vi "Teleop.vi"(10 "Match Info":T2={"Autonomous Elapsed Seconds"=0.0, "TeleOp Elapsed Seconds"=0.0, "Disabled Elapsed Seconds"=0.0, "Visited Autonomous"=FALSE, "Visited TeleOp"=FALSE, "Visited Disabled"=FALSE, "Autonomous Settings"={"Autonomous Style"=enum."Independent", "VI Refnum"=refnum}}, 11 "Call Context":T3) -> ()   [LabVIEW 2023]
doc: "This VI is called for each TeleOp packet received from the DS where the robot is not disabled. It is often used to read from the joysticks and update I/O or to update setpoints for timed control loops. It should complete and return within 20 milliseconds or it may miss DS packets."
uses:
  <vilib>/Rock Robotics/WPI/DriverStation/WPI_DriverStationDerivedRobotMode.ctl
  <vilib>/Rock Robotics/WPI/DriverStation/WPI_DriverStationMatch Info.ctl
  Shared Code/TypeDefs/ENUM_CMD_Mode Select.ctl
  Teleop Support/ENUM_Axes Select.ctl
  Systems/SwerveDrive/Cluster_CMD_ACT_Data.ctl
  Shared Code/TypeDefs/Cluster_CMD_Direction Data.ctl
  Shared Code/TypeDefs/Cluster_Module Velocity-Direction-Rotations.ctl
  Shared Code/TypeDefs/Level_Velocity plus-minus 1.ctl
  Shared Code/TypeDefs/Dial_Compase heading unit circle CCW positive.ctl
  Shared Code/TypeDefs/Cluster_X-Y.ctl
  8b3177bb-dc82-4863-aed5-aa104a122ccc.vi
  83fdd1ca-84e3-4cf5-86f5-8b3c56b849f5.vi
  <vilib>/Rock Robotics/Network Tables/NT Write Boolean.vi
  Systems/Game Controller/Global_SEN_Data Out.vi
  Systems/SwerveDrive/Global_CMD_ACT_Data In.vi
  Systems/Game Controller/GameController_SEN.lvlib
  Systems/SwerveDrive/SwerveDrive_ACT_ts.lvlib
panel:
  in  "MAx Traverse Speed FPS Out":dbl=5.0
  out "Drive Mode":T1
  out "POV":i16
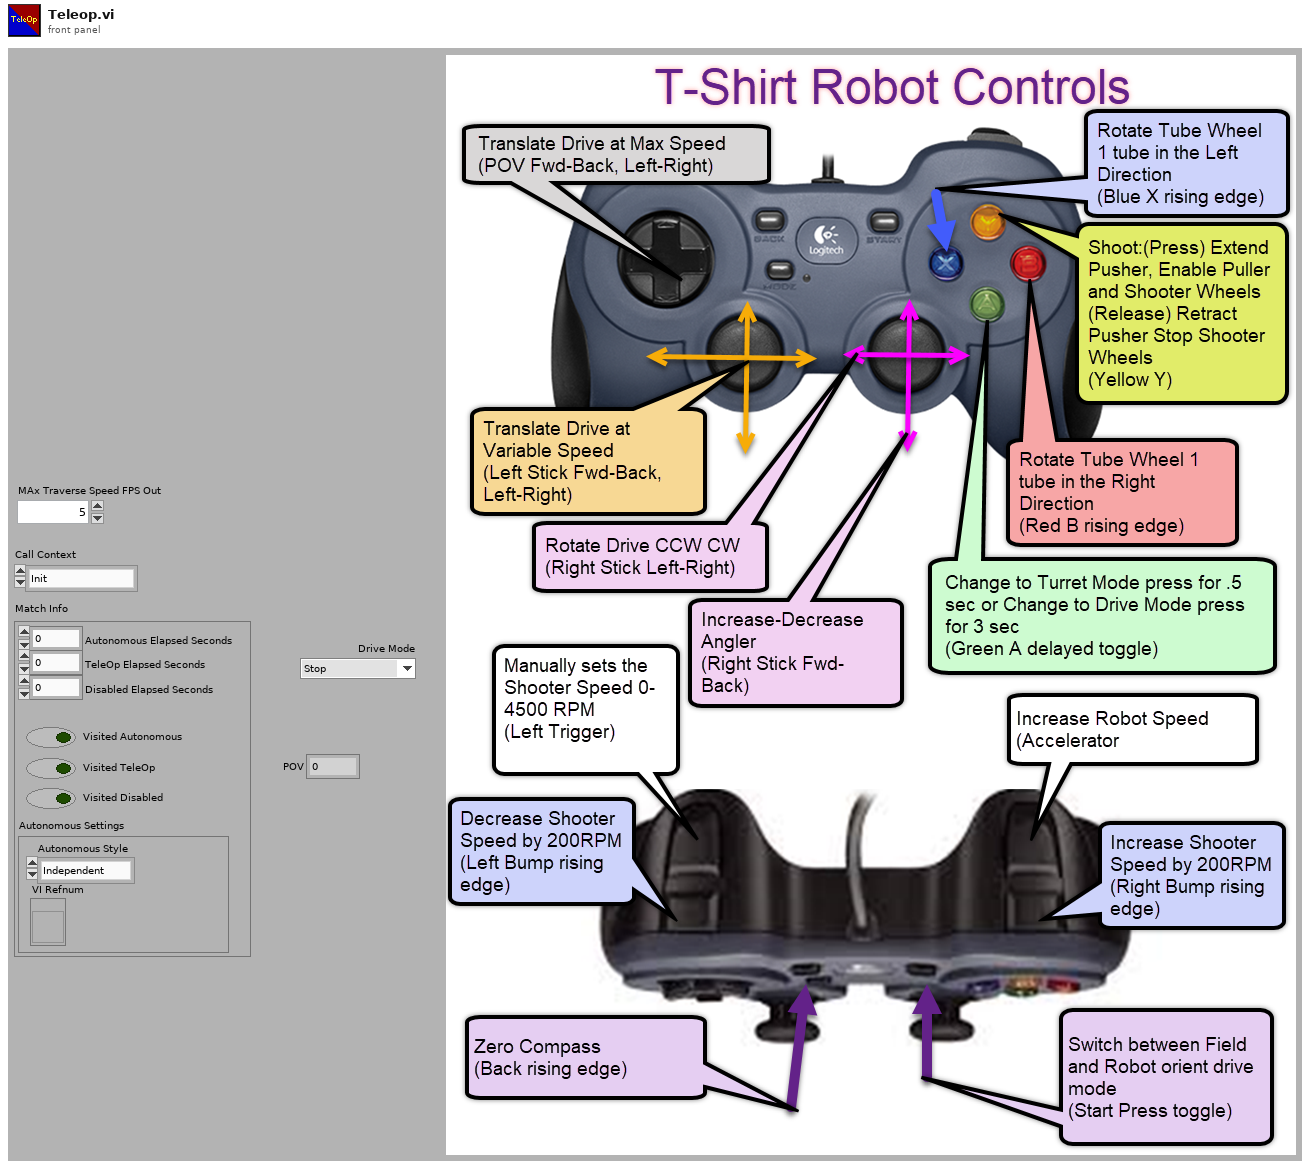
[diagram p1: front panel]
types:
  T1 = typedef "ENUM_CMD_Mode Select.ctl" = enum16{"Stop", "Move", "Turret Manual"}
  T2 = typedef "WPI_DriverStationMatch Info.ctl" = cluster{"Autonomous Elapsed Seconds":dbl, "TeleOp Elapsed Seconds":dbl, "Disabled Elapsed Seconds":dbl, "Visited Autonomous":bool, "Visited TeleOp":bool, "Visited Disabled":bool, "Autonomous Settings":cluster{"Autonomous Style":enum16{"Iterative", "Independent"}, "VI Refnum":refnum<vi>}}
  T3 = typedef "WPI_DriverStationDerivedRobotMode.ctl" = enum16{"Init", "Execute", "Stop"}
  T4 = typedef "ENUM_Axes Select.ctl" = enum16{"Left Stick Left (-1) Right (1)", "Left Stick Fwd (-1) Back(1)", "Left Trigger (0-1)", "Right Trigger (0-1)", "Right Stick Left(-1 Right (1)", "Right Stick Fwd(-1) Back (1)"}
  T5 = typedef "Cluster_Module Velocity-Direction-Rotations.ctl" = cluster{"Velocity":T6, "Angle":T7, "Rotations Count":dbl}
  T6 = typedef "Level_Velocity plus-minus 1.ctl" = dbl
  T7 = typedef "Dial_Compase heading unit circle CCW positive.ctl" = dbl
  T8 = typedef "SwerveDrive_ACT_ts.lvlib/Cluster_CMD_ACT_Data.ctl" = cluster{"Mode":T1, "Direction":T9, "Orientation Robot(t) Field(f)":bool, "Max Translation Speed (ft/sec)":dbl, "Rotation Reduction 1-0":dbl, "Rotation Center from Robot Center":T10, "Auto Angle":T7, "Auto Target (ft)":dbl}
  T9 = typedef "Cluster_CMD_Direction Data.ctl" = cluster{"Traverse":T5, "Rotate(Yaw) CCW 1 CW -1":dbl}
  T10 = typedef "Cluster_X-Y.ctl" = cluster{"X":dbl, "Y":dbl}
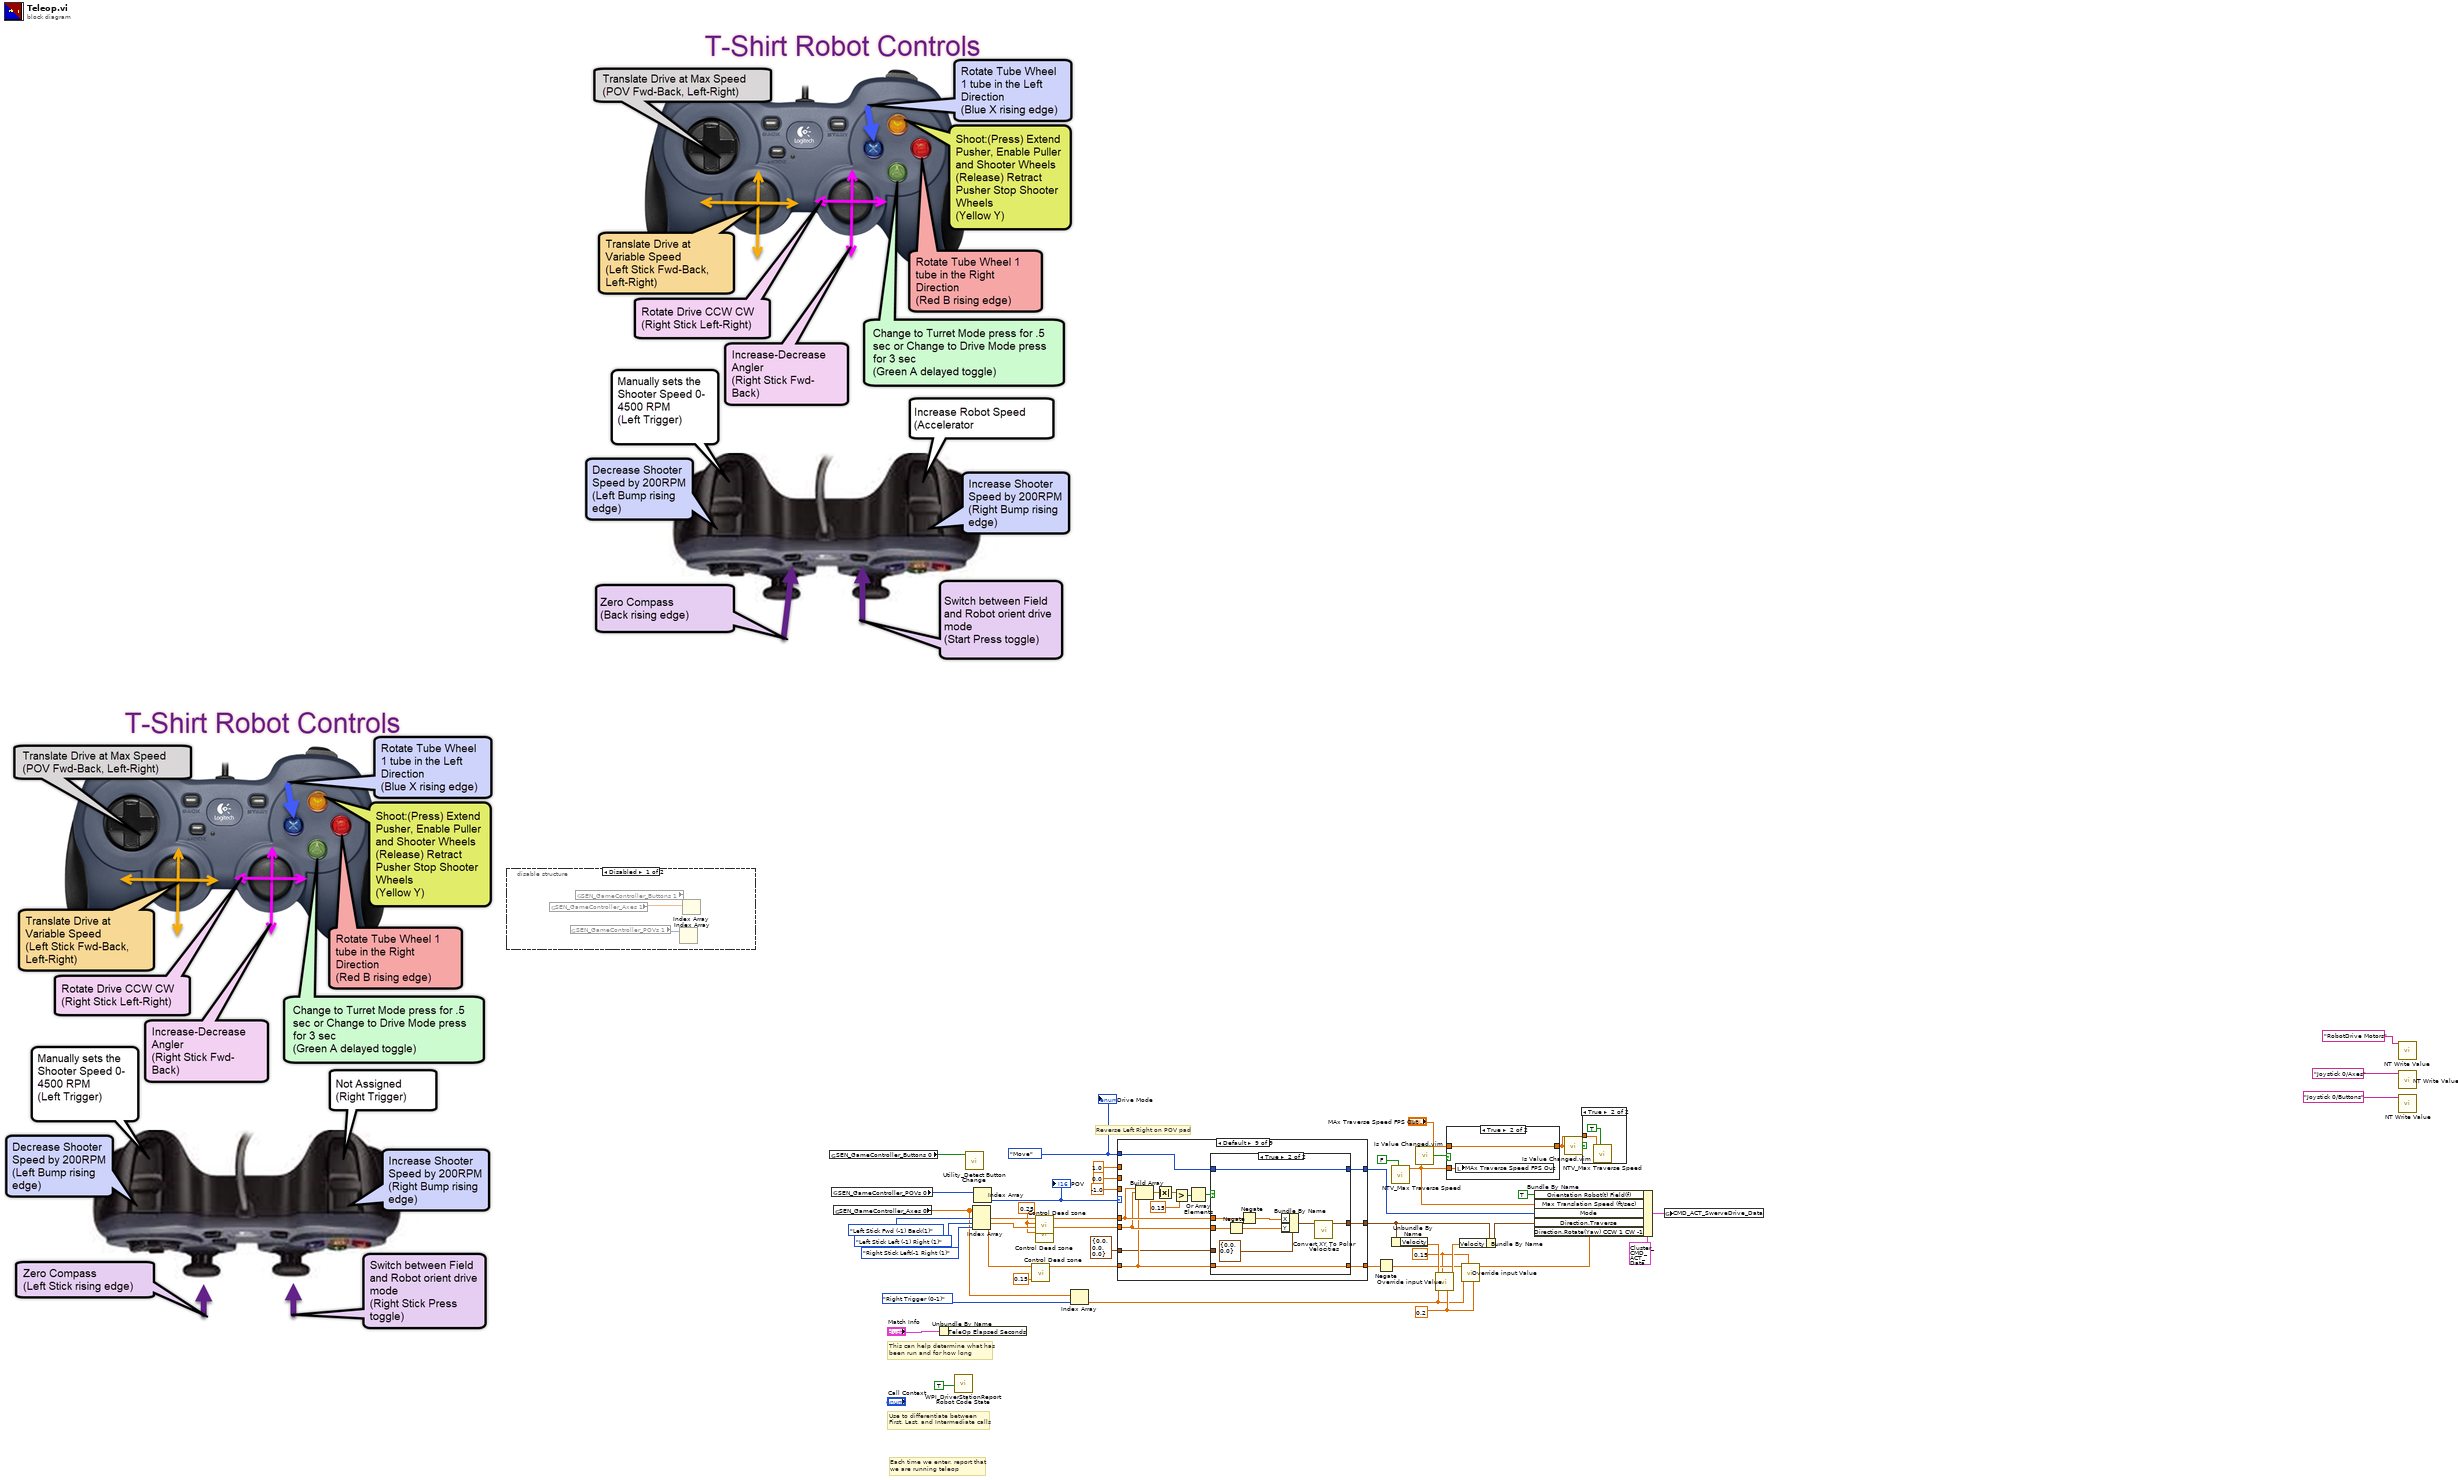
[diagram p0: block diagram]
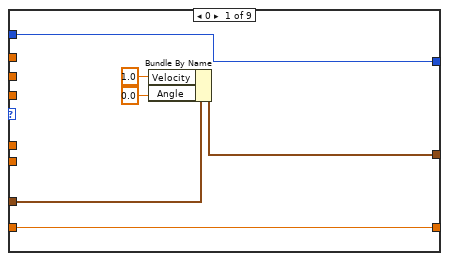
[diagram p5: hidden frame]
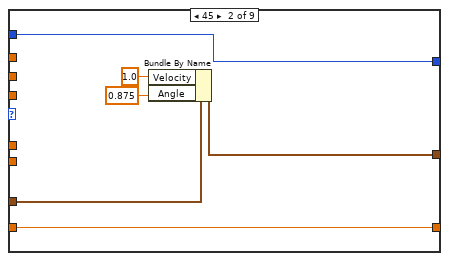
[diagram p6: hidden frame]
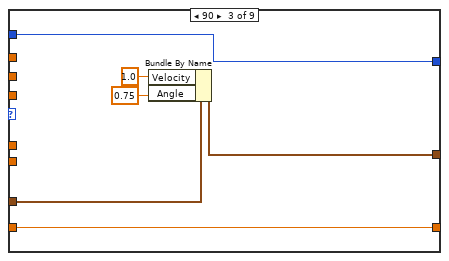
[diagram p7: hidden frame]
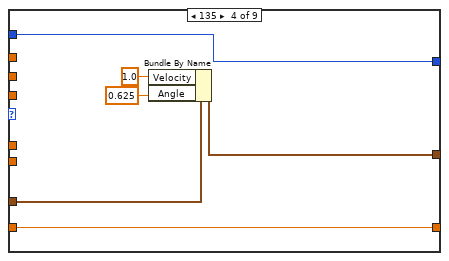
[diagram p8: hidden frame]
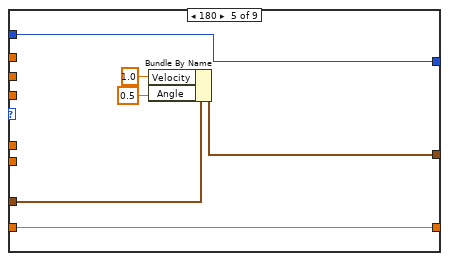
[diagram p9: hidden frame]
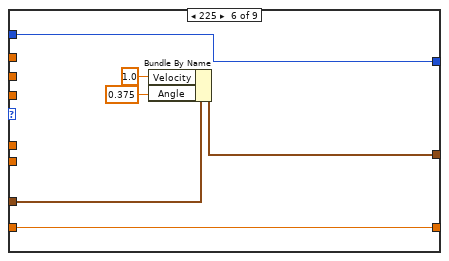
[diagram p10: hidden frame]
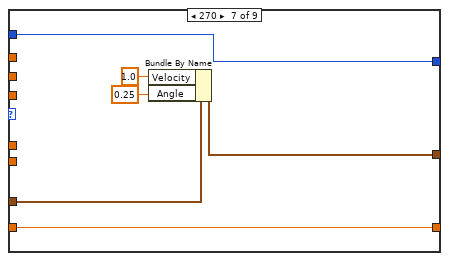
[diagram p11: hidden frame]
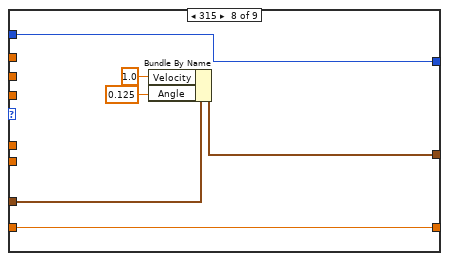
[diagram p12: hidden frame]
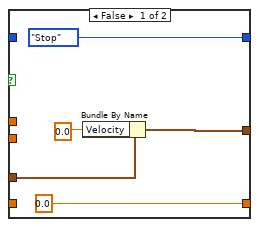
[diagram p13: hidden frame]
diagram:
  w22 = ENUM_CMD_Mode_Select."Move" ("Mode")
  w9 = 0.2 ("lower limit")
  w10 = 0.15 ("upper limit")
  w24 = 0.25 ("y")
  # "Reverse Left Right on POV pad"
  # "Each time we enter, report that\nwe are running teleop"
  # "Use to differentiate between\nFirst, Last, and Intermediate calls"
  # "This can help determine what has\nbeen run and for how long"
  n1 = disable-structure shown="Disabled" {
    frame Disabled {
      n2 = global read "Global_SEN_Data Out.vi" "SEN_GameController_Axes 1"() -> (w48:dbl[])
      n3 = global read "Global_SEN_Data Out.vi" "SEN_GameController_POVs 1"() -> (w47:i16[])
      n4 = global read "Global_SEN_Data Out.vi" "SEN_GameController_Buttons 1"() -> ()  [unwired: 1 out]
      n5 = Index Array(array=w47) -> ()  [unwired: 1 in, 1 out]
      n6 = Index Array(array=w48) -> ()  [unwired: 1 in, 1 out]
    }
    frame Enabled {
    }
  }
  n7 = global read "Global_SEN_Data Out.vi" "SEN_GameController_Buttons 0"() -> (w20:bool[])
  n8 = global read "Global_SEN_Data Out.vi" "SEN_GameController_POVs 0"() -> (w41:i16[])
  n9 = global read "Global_SEN_Data Out.vi" "SEN_GameController_Axes 0"() -> (w19:dbl[])
  n10 = Unbundle By Name("Match Info") -> ()  [unwired: 1 out]
  n11 = call <vilib>:"WPI_DriverStationReport Robot Code State.vi"("TeleOp"=TRUE ("Autonomous")) -> ()  [unwired: 10 in, 1 out]
  n12 = call "Utility_Detect Button Change.vi"("HW_Joystick_Buttons"=w20) -> ()  [unwired: 6 in, 5 out]
  n13 = Index Array(array=w19, index #1=ENUM_Axes_Select."Left Stick Fwd (-1) Back(1)" ("Axes Select"), index #2=ENUM_Axes_Select."Left Stick Left (-1) Right (1)" ("Axes Select"), index #3=ENUM_Axes_Select."Right Stick Left(-1 Right (1)" ("Axes Select")) -> (element #1=w30:dbl, element #2=w26:dbl, element #3=w25:dbl)
  n14 = Index Array(array=w41) -> (element=w38:i16)  [unwired: 1 in]
  "POV" <- w38
  n15 = call "Control Dead zone.vi"("dead zone"=0.15 ("y"), "control Value"=w25) -> ("output Value"=w17:dbl)  [unwired: 9 in]
  n16 = call "Control Dead zone.vi"("dead zone"=w24, "control Value"=w30) -> ("output Value"=w29:dbl)  [unwired: 9 in]
  n17 = call "Control Dead zone.vi"("dead zone"=w24, "control Value"=w26) -> ("output Value"=w27:dbl)  [unwired: 9 in]
  n18 = Index Array(array=w19, index=ENUM_Axes_Select."Right Trigger (0-1)" ("Axes Select")) -> (element=w8:dbl)
  n19 = case shown="Default" w38 {
    tunnel: 1.0 ("Direction.Travers Left 1 Right -1") -> [_ _ _ _ _ _ _ _ _]
    tunnel: 0.0 ("Direction.Travers Left 1 Right -1") -> [_ _ _ _ _ _ _ _ _]
    tunnel: -1.0 ("Direction.Travers Left 1 Right -1") -> [_ _ _ _ _ _ _ _ _]
    tunnel: w22 -> [w54 w60 w66 w72 w78 w84 w90 w96 w109]
    tunnel: [w54 w60 w66 w72 w78 w84 w90 w96 w108] -> w21
    tunnel: w29 -> [_ _ _ _ _ _ _ _ w106]
    tunnel: w27 -> [_ _ _ _ _ _ _ _ w105]
    tunnel: w17 -> [w53 w59 w65 w71 w77 w83 w89 w95 w104]
    tunnel: [w53 w59 w65 w71 w77 w83 w89 w95 w107] -> w31
    tunnel: T5 {"Velocity"=0.0, "Angle"=0.0, "Rotations Count"=0.0} ("Polar Out") -> [w52 w58 w64 w70 w76 w82 w88 w94 w98]
    tunnel: [w49 w55 w61 w67 w73 w79 w85 w91 w97] -> w15
    frame 0 {
      n20 = Bundle By Name(cluster=w52, "Velocity"=T6 1.0, "Angle"=T7 0.0) -> (w49:T5)
    }
    frame 45 {
      n21 = Bundle By Name(cluster=w58, "Velocity"=T6 1.0, "Angle"=T7 0.875) -> (w55:T5)
    }
    frame 90 {
      n22 = Bundle By Name(cluster=w64, "Velocity"=T6 1.0, "Angle"=T7 0.75) -> (w61:T5)
    }
    frame 135 {
      n23 = Bundle By Name(cluster=w70, "Velocity"=T6 1.0, "Angle"=T7 0.625) -> (w67:T5)
    }
    frame 180 {
      n24 = Bundle By Name(cluster=w76, "Velocity"=T6 1.0, "Angle"=T7 0.5) -> (w73:T5)
    }
    frame 225 {
      n25 = Bundle By Name(cluster=w82, "Velocity"=T6 1.0, "Angle"=T7 0.375) -> (w79:T5)
    }
    frame 270 {
      n26 = Bundle By Name(cluster=w88, "Velocity"=T6 1.0, "Angle"=T7 0.25) -> (w85:T5)
    }
    frame 315 {
      n27 = Bundle By Name(cluster=w94, "Velocity"=T6 1.0, "Angle"=T7 0.125) -> (w91:T5)
    }
    frame Default {
      n28 = Build Array(w106, w105, w104) -> (w103:dbl[])
      n29 = Absolute Value(x=w103) -> (abs(x)=w99:dbl[])
      n30 = Greater?(x=w99, y=0.15 ("upper limit")) -> (0:w101:bool[])
      n31 = Or Array Elements(Boolean array=w101) -> (logical OR=w100:bool)
      n32 = case shown="True" w100 {
        tunnel: w109 -> [_ w121]
        tunnel: [ENUM_CMD_Mode_Select."Stop" ("Mode") w121] -> w108
        tunnel: w106 -> [_ w123]
        tunnel: w105 -> [_ w122]
        tunnel: w104 -> [_ w120]
        tunnel: [0.0 ("f") w120] -> w107
        tunnel: w98 -> [w112 _]
        tunnel: [w113 w117] -> w97
        frame False {
          n33 = Bundle By Name(cluster=w112, "Velocity"=T6 0.0) -> (w113:T5)
        }
        frame True {
          n34 = Negate(x=w122) -> (-x=w116:dbl)
          n35 = Negate(x=w123) -> (-x=w115:dbl)
          n36 = Bundle By Name(cluster=T10 {"X"=0.0, "Y"=0.0} ("XY Velocities"), "X"=w115, "Y"=w116) -> (w119:T10)
          n37 = call "Convert XY To Polar Velocities.vi"("XY Velocities"=w119) -> ("Polar Out"=w117:T5)  [unwired: 10 in]
        }
      }
    }
  }
  n38 = Negate(x=w31) -> (-x=w12:dbl)
  n39 = call "NTV_Max Traverse Speed.vi"("Read(f) Write(t)"=FALSE) -> ("MAx Traverse Speed FPS Out"=w4:dbl)  [unwired: 10 in]
  n40 = Unbundle By Name(w15) -> ("Velocity"=w14:T6)
  n41 = call "Is Value Changed.vim"("value"=w4) -> ("changed or first call?"=w5:bool)
  n42 = call "Override input Value.vi"("Starting Override Value (0-1)"=w9, "Min Value To Overide (0-1)"=w10, "OverRide Value (0-1)"=w8, "Value In (0-1)"=w14) -> ("Value Out"=w13:T6)  [unwired: 7 in]
  n43 = case shown="True" w5 {
    tunnel: w4 -> [_ w126]
    tunnel: [w124 w125] -> w3
    tunnel: "MAx Traverse Speed FPS Out" -> [w124 w125]
    frame False {
    }
    frame True {
      n44 = local write "MAx Traverse Speed FPS Out"(w126) -> ()
    }
  }
  n45 = Bundle By Name(cluster=w15, "Velocity"=w13) -> (w16:T5)
  n46 = call "Override input Value.vi"("Starting Override Value (0-1)"=w9, "Min Value To Overide (0-1)"=w10, "OverRide Value (0-1)"=w8, "Value In (0-1)"=w12) -> ("Value Out"=w11:T6)  [unwired: 7 in]
  n47 = Bundle By Name(cluster=T8 {"Mode"=enum."Stop", "Direction"={"Traverse"={"Velocity"=0.0, "Angle"=0.0, "Rotations Count"=0.0}, "Rotate(Yaw) CCW 1 CW -1"=0.0}, "Orientation Robot(t) Field(f)"=FALSE, "Max Translation Speed (ft/sec)"=0.0, "Rotation Reduction 1-0"=0.0, "Rotation Center from Robot Center"={"X"=0.0, "Y"=0.0}, "Auto Angle"=0.0, "Auto Target (ft)"=0.0} ("CMD_ACT_Template_Data"), "Orientation Robot(t) Field(f)"=TRUE, "Max Translation Speed (ft/sec)"=w4, "Mode"=w21, "Direction.Traverse"=w16, "Direction.Rotate(Yaw) CCW 1 CW -1"=w11) -> (w33:T8)
  n48 = call "Is Value Changed.vim"("value"=w3) -> ("changed or first call?"=w6:bool)
  n49 = case shown="True" w6 {
    tunnel: w3 -> [_ w127]
    frame False {
    }
    frame True {
      n50 = call "NTV_Max Traverse Speed.vi"("Read(f) Write(t)"=TRUE, "MAx Tavers Speed FPS"=w127) -> ()  [unwired: 9 in, 1 out]
    }
  }
  n51 = global write "Global_CMD_ACT_Data In.vi" "CMD_ACT_SwerveDrive_Data"(w33) -> ()
  n52 = call-poly <vilib>:"NT Write Value.vi"("name"="RobotDrive Motors" ("Name")) -> ()  [unwired: 10 in, 1 out]
  n53 = call-poly <vilib>:"NT Write Value.vi"("name"="Joystick 0/Axes" ("Name")) -> ()  [unwired: 10 in, 1 out]
  n54 = call-poly <vilib>:"NT Write Value.vi"("name"="Joystick 0/Buttons" ("Name")) -> ()  [unwired: 10 in, 1 out]
  "Drive Mode" <- w22
